vi "PH_Beckhoff_Application.declare digital MA01 OutputTags.vi"() -> (0 "Digital Outputs":T2, 1 "Description":string)   [LabVIEW 2014, in "PH_Beckhoff_Application.lvlib"]
uses:
  PH_Beckhoff_Application.lvlib
  PH_Beckhoff/PH_Beckhoff.Digital Outputs.ctl
  PH_Beckhoff/PH_Beckhoff.lvlib
panel:
  in  "Digital Output Value":T1
  out "Right Size?":bool
  # "Let this VI run to check the size!"
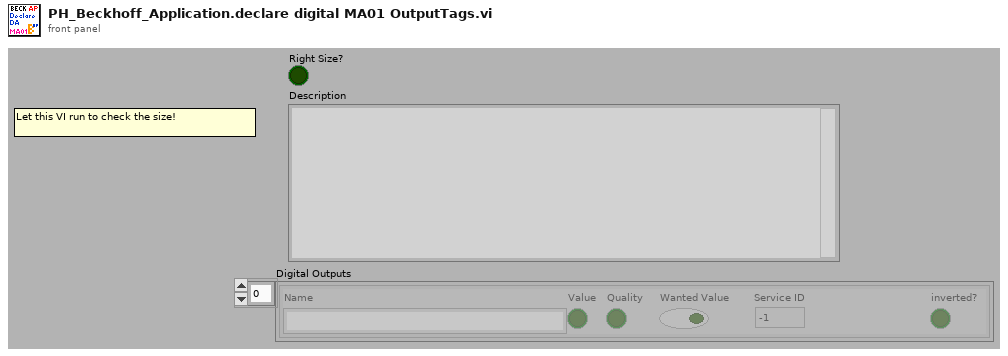
[diagram p1: front panel]
types:
  T1 = cluster{"Name":string, "Value":bool, "Quality":bool, "Wanted Value":bool, "Service ID":i32, "inverted?":bool}
  T2 = typedef "PH_Beckhoff.lvlib/PH_Beckhoff.Digital Outputs.ctl" = cluster{"Name":string, "Value":bool, "Quality":bool, "Wanted Value":bool, "Service ID":i32, "inverted?":bool}[]
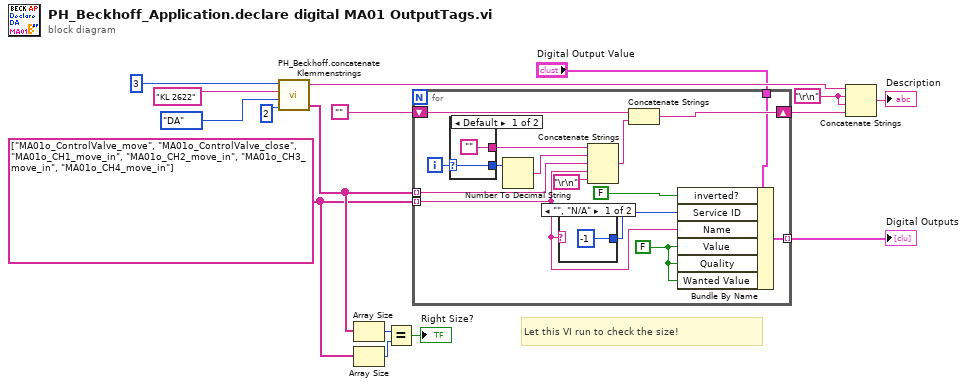
[diagram p0: block diagram]
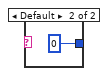
[diagram p2: hidden frame]
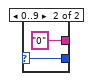
[diagram p3: hidden frame]
diagram:
  w3 = string[] ["MA01o_ControlValve_move", "MA01o_ControlValve_close", "MA01o_CH1_move_in", "MA01o_CH2_move_in", "MA01o_CH3_move_in", "MA01o_CH4_move_in"] ("appended array")
  w13 = "\r\n"
  # "Let this VI run to check the size!"
  n1 = call "PH_Beckhoff.concatenate Klemmenstrings.vi"("# of In- or Outputs"=2, "Type"=enum16{"AE", "AA", "DE", "DA"}."DA", "Klemmenname"="KL 2622", "Quantity"=3 ("size(s)")) -> ("concatenated string array"=w5:string[], "\"<Type>: <Quantity> x <Klemmenname>\""=w4:string)  [unwired: 1 out]
  n2 = Array Size(array=w5) -> (size(s)=w9:i32)
  n3 = Array Size(array=w3) -> (size(s)=w8:i32)
  n4 = Equal?(x=w9, y=w8) -> (x = y?=→"Right Size?":bool)
  n5 = for {
    tunnel: w3 -> [w20] mode=indexing
    tunnel: w5 -> [w27] mode=indexing
    shift-right: [w24] -> w14
    shift-left: "" -> [w23]
    tunnel: "Digital Output Value" -> [w18]
    tunnel: [w17] -> w1 mode=indexing
    i -> [w31]
    w19 = FALSE ("Quality")
    n6 = case shown="Default" w31 {
      selector: w31 -> [w34 w37]
      tunnel: [w34 w37] -> w30
      tunnel: ["" "0"] -> w29
      frame Default {
      }
      frame 0..9 {
      }
    }
    n7 = Number To Decimal String(number=w30) -> (decimal integer string=w28:string)  [unwired: 1 in]
    n8 = case shown="\"\", \"N/A\"" w20 {
      tunnel: [-1 0] -> w21
      frame "", "N/A" {
      }
      frame Default {
      }
    }
    n9 = Concatenate Strings(w29, w28, w27, w20, "\r\n") -> (w25:string)
    n10 = Concatenate Strings(w23, w25) -> (w24:string)
    n11 = Bundle By Name(cluster=w18, "inverted?"=FALSE, "Service ID"=w21, "Name"=w20, "Value"=w19, "Quality"=w19, "Wanted Value"=w19) -> (w17:T1)
  }
  "Digital Outputs" <- w1
  n12 = Concatenate Strings(w4, w13, w13, w14) -> (→"Description":string)
